vi "Wait for Tigger.vi"(8 "error in (no error)":errorcluster, 11 "rfsa queue":refnum<queue>) -> (0 "error out":errorcluster, 3 "abort?":bool)   [LabVIEW 2021]
uses:
  RFSA Configuration.ctl
  Messaging/RFSA Message.ctl
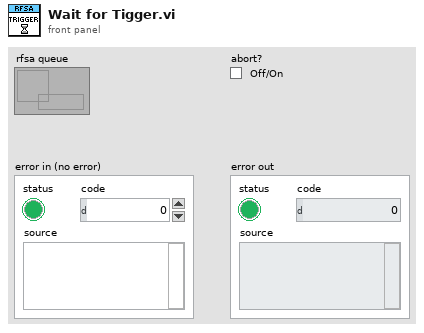
[diagram p1: front panel]
types:
  T1 = typedef "RFSA Message.ctl" = enum16{"Trigger Ready", "Run RF", "Stop RF", "Exit"}
  T2 = typedef "RFSA Configuration.ctl" = cluster{"rfsa ref":refnum<k15>, "cent freq":dbl, "iq rate":dbl, "power":dbl, "N/block":i64, "msg":T1}
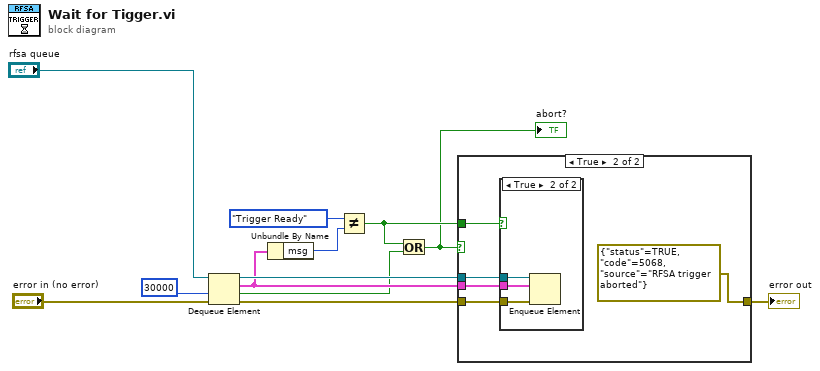
[diagram p0: block diagram]
diagram:
  n1 = Dequeue Element(queue="rfsa queue", timeout in ms (-1)=30000, error in (no error)="error in (no error)") -> (queue out=w9:refnum<queue>, element=w8:T2, timed out?=w7:bool, error out=w10:errorcluster)
  n2 = Unbundle By Name(w8) -> ("msg"=w11:T1)
  n3 = Not Equal?(x=RFSA_Message."Trigger Ready", y=w11) -> (x != y?=w2:bool)
  n4 = Or(x=w2, y=w7) -> (x .or. y?=w1:bool)
  "abort?" <- w1
  n5 = case shown="True" w1 {
    tunnel: w10 -> [w13 w18]
    tunnel: [w13 errorcluster {"status"=TRUE, "code"=5068, "source"="RFSA trigger aborted"} ("error out")] -> w6
    tunnel: w9 -> [_ w17]
    tunnel: w8 -> [_ w16]
    tunnel: w2 -> [_ w14]
    frame False {
    }
    frame True {
      n6 = case shown="True" w14 {
        tunnel: w18 -> [_ w21]
        tunnel: w17 -> [_ w20]
        tunnel: w16 -> [_ w19]
        frame False {
        }
        frame True {
          n7 = Enqueue Element(queue=w20, element=w19, error in (no error)=w21) -> ()  [unwired: 1 in, 3 out]
        }
      }
    }
  }
  "error out" <- w6
